vi "DataSetReferencesToData.vi"(8 "error in (no error)":errorcluster, 11 "data event":T1) -> (0 "error out":errorcluster, 3 "data event out":T1)   [LabVIEW 2017, in "FileManager.lvlib"]
uses:
  <vilib>/addons/InsightCM/Devices/Shared/Common/FileManager/FileManager.lvlib
  <vilib>/addons/InsightCM/Devices/Shared/Common/DataEvent/controls/Event.ctl
  <vilib>/addons/InsightCM/MessageBus/Base/controls/DataEvent.ctl
  <vilib>/addons/InsightCM/MessageBus/Base/controls/KeyValuePair.ctl
  <vilib>/addons/InsightCM/Devices/Shared/Common/DataEvent/controls/DataSet.ctl
  <vilib>/addons/InsightCM/MessageBus/Base/controls/DataSetMetadata.ctl
  <vilib>/addons/InsightCM/MessageBus/Base/controls/TrendPoint.ctl
  <vilib>/addons/InsightCM/MessageBus/Base/controls/TrendAlarmUpdate.ctl
  <vilib>/addons/InsightCM/MessageBus/Base/controls/TrendAlarmTransition.ctl
  <vilib>/addons/InsightCM/Devices/Shared/Common/DataEventCreator/DataEventCreator.lvlib
  <vilib>/addons/InsightCM/Devices/Shared/Common/DataEvent/DataEvent.lvlib
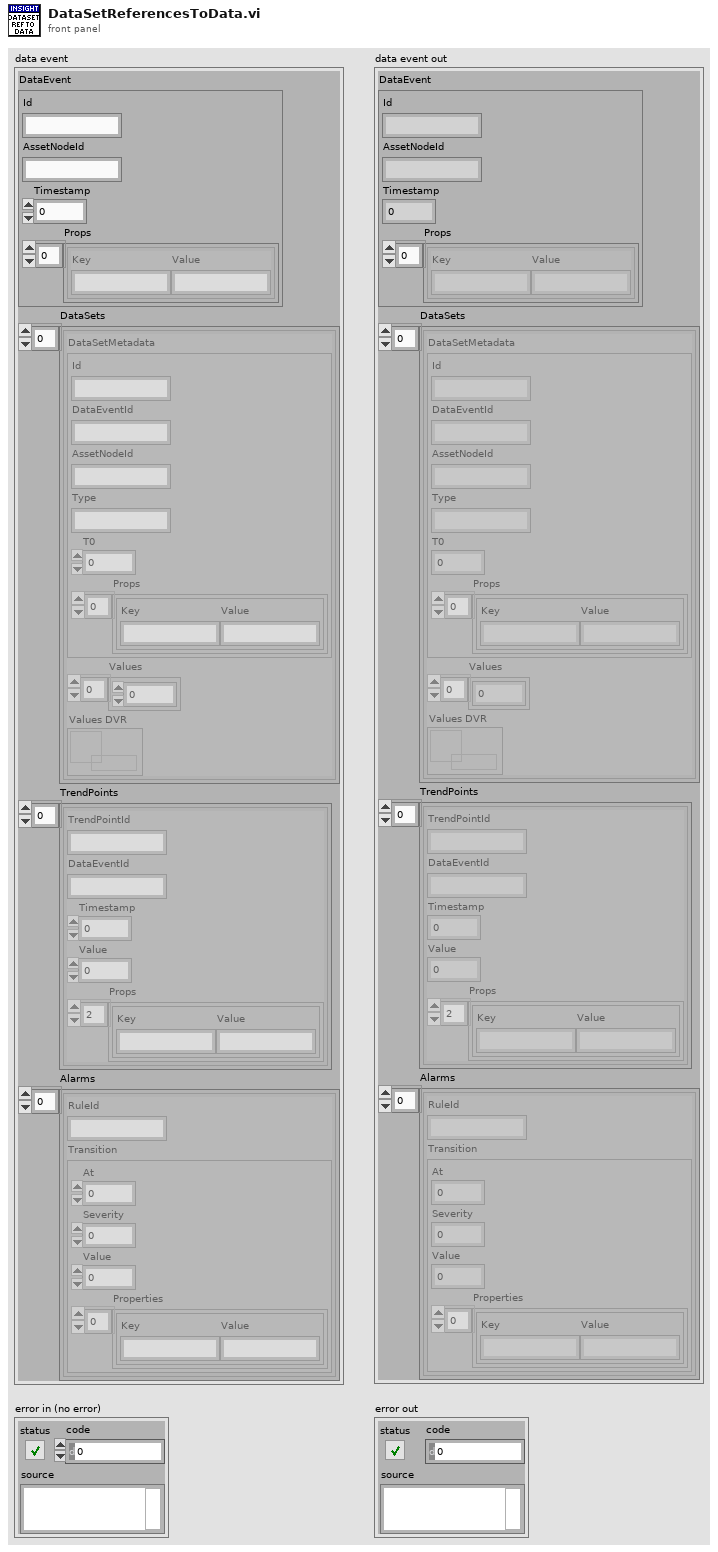
[diagram p1: front panel]
types:
  T1 = typedef "DataEvent.lvlib/Event.ctl" = cluster{"DataEvent":T2, "DataSets":T4[], "TrendPoints":T6[], "Alarms":T7[]}
  T2 = typedef "DataEvent.ctl" = cluster{"Id":string, "AssetNodeId":string, "Timestamp":i64, "Props":T3[]}
  T3 = typedef "KeyValuePair.ctl" = cluster{"Key":string, "Value":string}
  T4 = typedef "DataEvent.lvlib/DataSet.ctl" = cluster{"DataSetMetadata":T5, "Values":sgl[], "Values DVR":refnum<data-value>}
  T5 = typedef "DataSetMetadata.ctl" = cluster{"Id":string, "DataEventId":string, "AssetNodeId":string, "Type":string, "T0":i64, "Props":T3[]}
  T6 = typedef "TrendPoint.ctl" = cluster{"TrendPointId":string, "DataEventId":string, "Timestamp":i64, "Value":dbl, "Props":T3[]}
  T7 = typedef "TrendAlarmUpdate.ctl" = cluster{"RuleId":string, "Transition":T8}
  T8 = typedef "TrendAlarmTransition.ctl" = cluster{"At":i64, "Severity":i32, "Value":dbl, "Properties":T3[]}
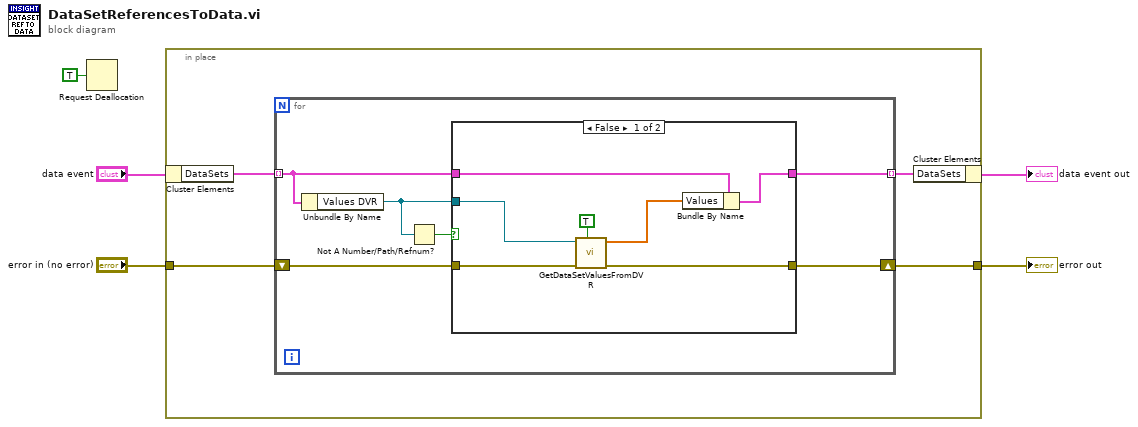
[diagram p0: block diagram]
diagram:
  n1 = Request Deallocation(TRUE ("flag")) -> ()
  n2 = in-place {
    in-place-border: "error in (no error)" -> [w7]
    in-place-border: [w6] -> w3
    n3 = in-place-cluster #1("data event") -> ("DataSets"=w9:T4[])
    n4 = for {
      tunnel: w9 -> [w11] mode=indexing
      tunnel: [w12] -> w8 mode=indexing
      shift-right: [w10] -> w6
      shift-left: w7 -> [w15]
      n5 = Unbundle By Name(w11) -> ("Values DVR"=w13:refnum<data-value>)
      n6 = Not A Number/Path/Refnum?(number/path/refnum=w13) -> (NaN/Path/Refnum?=w14:bool)
      n7 = case shown="False" w14 {
        tunnel: w15 -> [w21 w23]
        tunnel: w13 -> [w20 _]
        tunnel: [w16 w24] -> w12
        tunnel: w11 -> [w18 w24]
        tunnel: [w19 w23] -> w10
        frame False {
          n8 = call <vilib>:"GetDataSetValuesFromDVR.vi"("delete dvr"=TRUE, "error in (no error)"=w21, "values dvr"=w20) -> ("error out"=w19:errorcluster, "values"=w17:sgl[])  [unwired: 7 in]
          n9 = Bundle By Name(cluster=w18, "Values"=w17) -> (w16:T4)
        }
        frame True {
        }
      }
    }
    n10 = in-place-cluster #1("DataSets"=w8) -> (→"data event out":T1)
  }
  "error out" <- w3
